vi "_SHARED_TXT-Savedata_SingleCh.vi"(5 "Arraych6":dbl[](array[numeric]), 7 "Array Time":timestamp[](array[timestamp]), 8 "error in (no error)":errorcluster, 10 "Suffisso":string, 11 "file path (use dialog)":path) -> (0 "error out":errorcluster, 3 "LastSaved":string)   [LabVIEW 2020]
panel:
  in  "Name array acq":string="LC[kN]"
  in  "Name array Time":string="TIME"
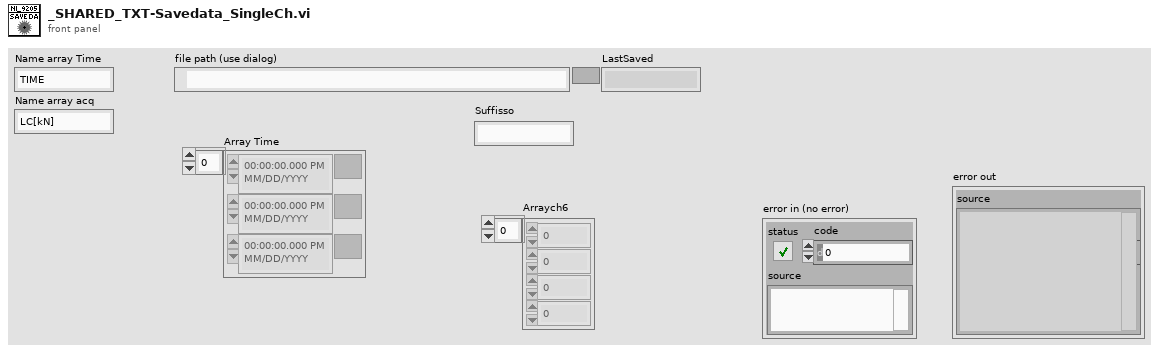
[diagram p1: front panel]
types:
  T1 = enum16{"open", "replace", "create", "open or create", "replace or create", "replace or create with confirmation"}
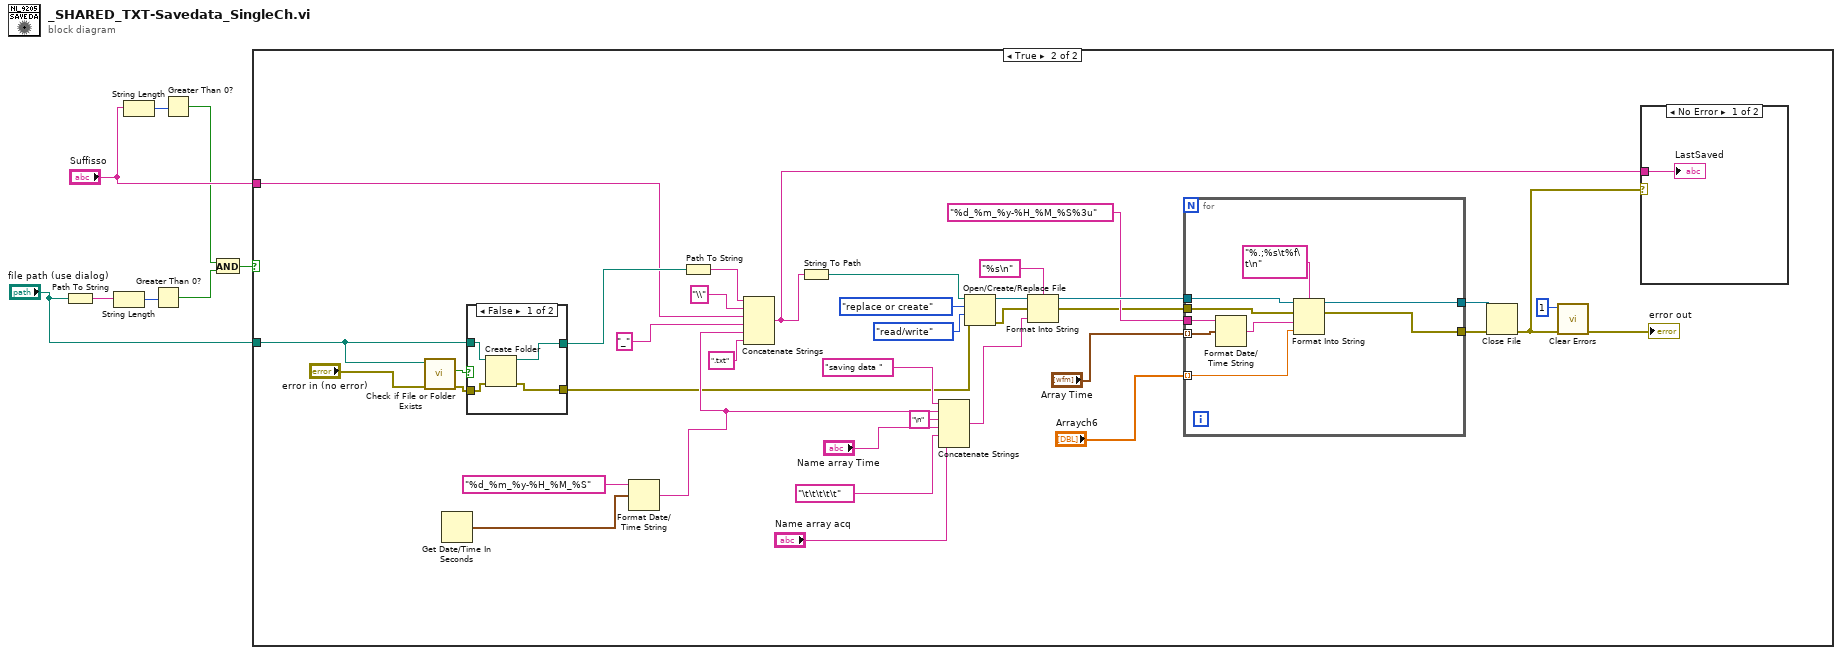
[diagram p0: block diagram]
diagram:
  n1 = Path To String(path="file path (use dialog)") -> (string=w4:string)
  n2 = String Length(string=w4) -> (length=w6:i32)
  n3 = String Length(string="Suffisso") -> (length=w7:i32)
  n4 = Greater Than 0?(x=w6) -> (x > 0?=w3:bool)
  n5 = Greater Than 0?(x=w7) -> (x > 0?=w2:bool)
  n6 = And(x=w2, y=w3) -> (x .and. y?=w1:bool)
  n7 = case shown="True" w1 {
    tunnel: "Suffisso" -> [_ w17]
    tunnel: "file path (use dialog)" -> [_ w12]
    frame False {
    }
    frame True {
      n8 = call <vilib>:"Check if File or Folder Exists.vi"("error in (no error)"="error in (no error)", "path"=w12) -> ("error out"=w19:errorcluster, "file or folder exists?"=w21:bool)  [unwired: 7 in, 1 out]
      n9 = Get Date/Time In Seconds() -> (seconds since 1Jan1904=w31:timestamp)
      n10 = case shown="False" w21 {
        tunnel: [w50 w52] -> w25
        tunnel: w19 -> [w47 w52]
        tunnel: w12 -> [w49 w51]
        tunnel: [w48 w51] -> w18
        frame False {
          n11 = Create Folder(path (use dialog)=w49, error in=w47) -> (created path=w48:path, error out=w50:errorcluster)  [unwired: 1 in, 1 out]
        }
        frame True {
        }
      }
      n12 = Format Date/Time String(time format string (%c)="%d_%m_%y-%H_%M_%S", seconds (now)=w31) -> (date/time string=w30:string)  [unwired: 1 in]
      n13 = Path To String(path=w18) -> (string=w35:string)
      n14 = Concatenate Strings(w35, "\\" ("string"), w17, "_" ("string"), w30, ".txt" ("string")) -> (w16:string)
      n15 = String To Path(string=w16) -> (path=w29:path)
      n16 = Concatenate Strings("saving data ", w30, "\n" ("string"), "Name array Time", "\t\t\t\t\t" ("string"), "Name array acq") -> (w38:string)
      n17 = Open/Create/Replace File(file path (use dialog)=w29, error in=w25, operation (0:open)=T1."replace or create", access (0:read/write)=enum16{"read/write", "read-only", "write-only"}."read/write") -> (refnum out=w41:refnum<file>, error out=w24:errorcluster)  [unwired: 2 in, 1 out]
      n18 = Format Into String(format string="%s\n", initial string=w41, error in=w24, w38) -> (resulting string=w36:refnum<file>, error out=w23:errorcluster)
      n19 = for {
        tunnel: w36 -> [w61]
        tunnel: "Arraych6" -> [w55] mode=indexing
        tunnel: [w59] -> w42
        tunnel: "%d_%m_%y-%H_%M_%S%3u" ("time format string (%c)") -> [w58]
        tunnel: "Array Time" -> [w57] mode=indexing
        tunnel: w23 -> [w54]
        tunnel: [w53] -> w22
        n20 = Format Date/Time String(time format string (%c)=w58, seconds (now)=w57) -> (date/time string=w56:string)  [unwired: 1 in]
        n21 = Format Into String(format string="%.;%s\t%f\t\n", initial string=w61, error in=w54, w56, w55) -> (resulting string=w59:refnum<file>, error out=w53:errorcluster)
      }
      n22 = Close File(refnum=w42, error in=w22) -> (error out=w13:errorcluster)  [unwired: 1 out]
      n23 = call <vilib>:"Clear Errors.vi"("error in (no error)"=w13, "specific error code to clear (0: all)"=1) -> ("error out"=→"error out":errorcluster)  [unwired: 4 in, 1 out]
      n24 = case shown="No Error" w13 {
        tunnel: w16 -> [w46 _]
        frame No Error {
          "LastSaved" <- w46
        }
        frame Error {
        }
      }
    }
  }
